vi "Terminate control (SubVI).vi"(8 "errorin":errorcluster) -> (0 "error out":errorcluster)   [LabVIEW 2016]
uses:
  <vilib>/Utility/sysdir.llb/System Directory Type.ctl
  <vilib>/Utility/config.llb/Write Key (String).vi
  <vilib>/Utility/config.llb/NI_LVConfig.lvlib
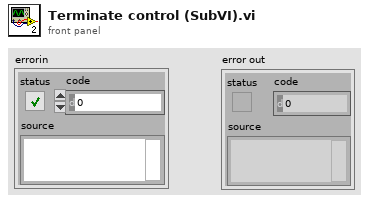
[diagram p1: front panel]
types:
  T1 = typedef "System Directory Type.ctl" = i32
  T2 = typedef "NI_LVConfig.lvlib/Config Data RefNum.ctl" = refnum<k1>
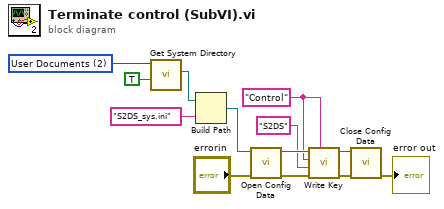
[diagram p0: block diagram]
diagram:
  w6 = "Control" ("section")
  w9 = T1 2 items=["User Home"=0, "User Desktop"=1, "User Documents"=2, "User Application Data"=3, "User Preferences"=4, "User Temporary"=5, "Public Documents"=6, "Public Application Data"=7, "Public Preferences"=8, "Public Cache"=13, "System Core Libraries"=9, "System Installed Libraries"=10, "Application Files"=11, "Boot Volume Root"=12] ("system directory type")
  n1 = call <vilib>:"Get System Directory.vi"("create directory if not found? (F)"=TRUE, "system directory type"=w9) -> ("system directory"=w1:path)  [unwired: 9 in]
  n2 = Build Path(base path=w1, name or relative path="S2DS_sys.ini") -> (appended path=w8:path)
  n3 = call <vilib>:"Open Config Data.vi"("error in (no error)"="errorin", "configuration file path"=w8) -> ("error out"=w5:errorcluster, "refnum"=w7:T2)  [unwired: 7 in, 1 out]
  n4 = call-poly <vilib>:"Write Key.vi"("section"=w6, "error in (no error)"=w5, "value"="S2DS", "key"=w6, "refnum"=w7) -> ("error out"=w3:errorcluster, "refnum out"=w4:T2)  [unwired: 4 in, 1 out]
  n5 = call <vilib>:"Close Config Data.vi"("error in (no error)"=w3, "refnum"=w4) -> ("error out"=→"error out":errorcluster)  [unwired: 8 in, 1 out]
